vi "Inst.Xeryon-Rotator.Stop.vi"(8 "error in (no error)":errorcluster, 11 "Inst.Xeryon-Rotator in":refnum<class "Inst.Xeryon-Rotator.lvclass">) -> (0 "error out":errorcluster, 3 "Inst.Xeryon-Rotator out":refnum<class "Inst.Xeryon-Rotator.lvclass">)   [LabVIEW 2019, in "Inst.Xeryon-Rotator.lvclass"]
uses:
  Inst.Xeryon-Rotator.lvclass
  Inst.Xeryon-Rotator.lvclass/Inst.Xeryon-Rotator.ctl
  Controller.LV/Controller.LV.lvclass
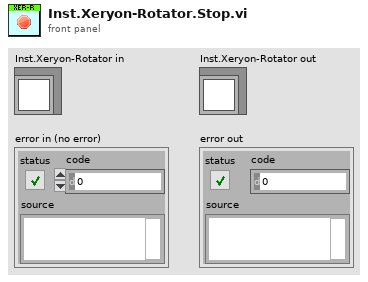
[diagram p1: front panel]
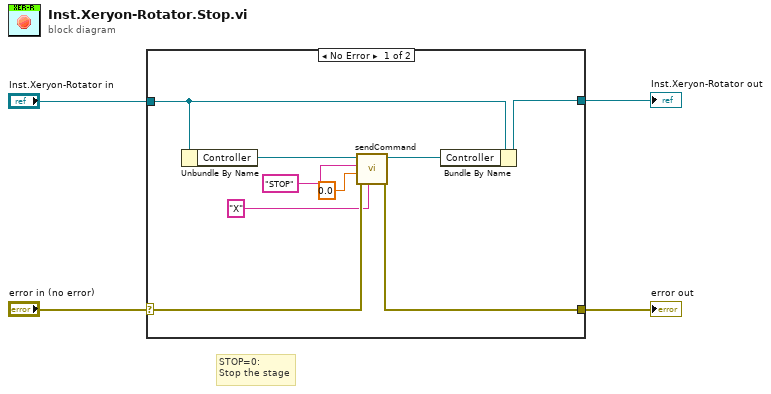
[diagram p0: block diagram]
diagram:
  # "STOP=0:\nStop the stage"
  n1 = case shown="No Error" "error in (no error)" {
    selector: "error in (no error)" -> [w8 w15]
    tunnel: [w13 w14] -> w1
    tunnel: [w10 w15] -> w2
    tunnel: "Inst.Xeryon-Rotator in" -> [w9 w14]
    frame No Error {
      n2 = Unbundle By Name(w9) -> ("Controller"=w12:refnum<class "Controller.LV.lvclass">)
      n3 = call-dynamic "sendCommand.vi"("Axis Letter"="X", "error in (no error)"=w8, "Value"=0.0, "Command"="STOP", "Controller in"=w12) -> ("error out"=w10:errorcluster, "Controller out"=w11:refnum<class "Controller.LV.lvclass">)  [unwired: 5 in]
      n4 = Bundle By Name(cluster=w9, "Controller"=w11) -> (w13:refnum<class "Inst.Xeryon-Rotator.lvclass">)
    }
    frame Error {
    }
  }
  "error out" <- w2
  "Inst.Xeryon-Rotator out" <- w1
